vi "NI VeriStand - Run Stimulus Profile.vi"(4 "Custom Model Parameter Files":path[](array[path]), 5 "Stop Stimulus Profile on Disconnect (T)":bool=TRUE, 6 "Timeout (120000 ms)":u32=120000, 7 "Autostart Stimulus Profile (T)":bool=TRUE, 8 "error in (no error)":errorcluster, 9 "Logging Directory Base Path":path, 10 "Stimulus Profile File":path, 11 "StimulusProfileManager in":T1) -> (0 "error out":errorcluster, 3 "StimulusProfileManager out":T1)   [LabVIEW 2020, in "NI_VS Stimulus ExecutionAPI.lvlib"]
doc: "This VI interfaces with the legacy Stimulus Profile Editor workspace tool in NI VeriStand, and is included for compatibility only. National Instruments recommends you use the current Stimulus Profile VIs to create, observe, and control NI VeriStand stimulus profiles and real-time sequences.\n\nRuns a stimulus profile file and logs data to a TDMS file in the directory you specify."
uses:
  <vilib>/NI VeriStand/Execution/Stimulus/NI_VS Stimulus ExecutionAPI.lvlib
  <vilib>/NI VeriStand/Execution/Stimulus/StimulusAPI.ctl
  NationalInstruments.VeriStand.ClientAPI
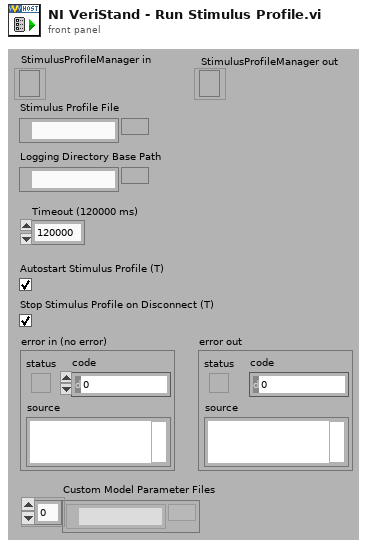
[diagram p1: front panel]
types:
  T1 = typedef "NI_VS Stimulus ExecutionAPI.lvlib/StimulusAPI.ctl" = refnum<k24>
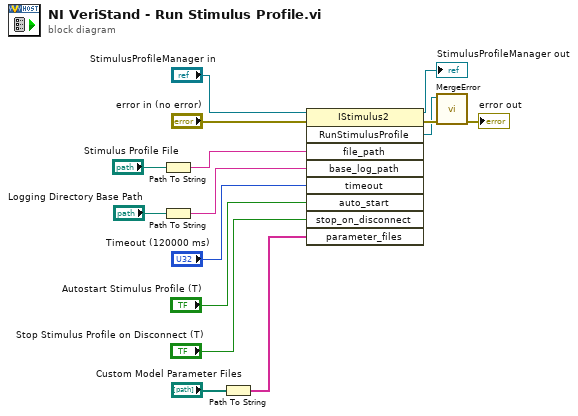
[diagram p0: block diagram]
diagram:
  n1 = Path To String(path="Stimulus Profile File") -> (string=w10:string)
  n2 = Path To String(path="Logging Directory Base Path") -> (string=w8:string)
  n3 = Path To String(path="Custom Model Parameter Files") -> (string=w1:string[])
  n4 = invoke class="IStimulus2" method="RunStimulusProfile"(reference="StimulusProfileManager in", error in="error in (no error)", "file_path"=w10, "base_log_path"=w8, "timeout"="Timeout (120000 ms)", "auto_start"="Autostart Stimulus Profile (T)", "stop_on_disconnect"="Stop Stimulus Profile on Disconnect (T)", "parameter_files"=w1) -> (reference out=→"StimulusProfileManager out":T1, error out=w15:errorcluster, "RunStimulusProfile"=w13:refnum<k24>)  [unwired: 1 in, 6 out]
  n5 = call <vilib>:"MergeError.vi"("error in (no error)"=w15, "Error"=w13) -> ("error out"=→"error out":errorcluster)  [unwired: 9 out]
